vi "Temperature Limit.vi"(3 "High Limit":dbl=80.0 format="%.2f", 4 "delta t (ms)":u32=400 min=50 max=2000 step=50, 5 "Points to Acquire":i32=75 min=20 max=500) -> ()   [LabVIEW 2010]
doc: "This VI simulates the acquisition of temperature, graphs the temperature, and notifies the user if the temperature is over the limit."
panel:
  out "Over Limit":bool
  in  "Abort":bool
  out "Temperature":cluster{"Temperature":dbl, "High Limit":dbl}(graph)
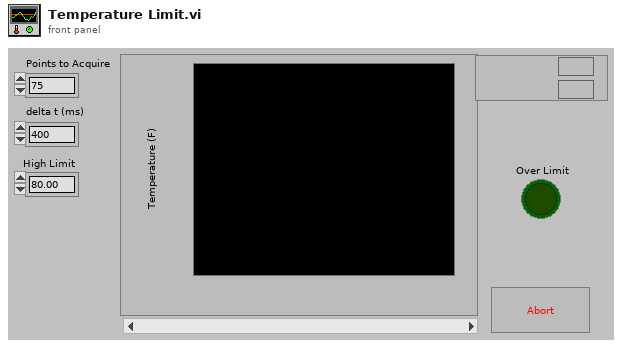
[diagram p1: front panel]
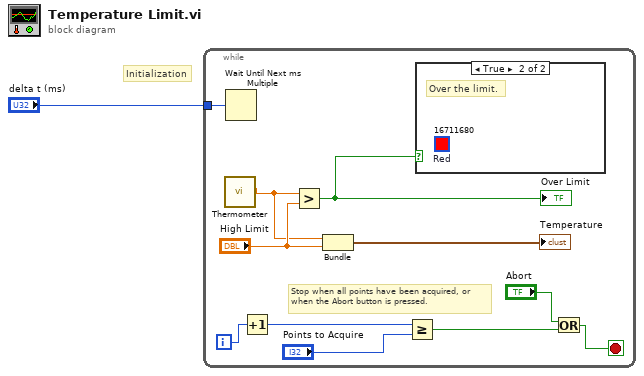
[diagram p0: block diagram]
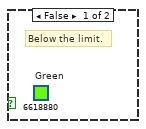
[diagram p2: hidden frame]
diagram:
  # "Initialization"
  n1 = while {
    tunnel: "delta t (ms)" -> [w4]
    i -> [w11]
    stop <- w5 stop-if-true
    # "Stop when all points have been acquired, or when the Abort button is pressed."
    n2 = call "Thermometer.vi"() -> ("Temperature"=w2:dbl)  [unwired: 10 in, 1 out]
    n3 = Wait Until Next ms Multiple(millisecond multiple=w4) -> ()  [unwired: 1 out]
    n4 = Increment(x=w11) -> (x+1=w9:i32)
    n5 = Greater?(x=w2, y="High Limit") -> (0:w3:bool)
    "Over Limit" <- w3
    n6 = Bundle("Temperature"=w2, "High Limit"="High Limit") -> (→"Temperature":cluster{"Temperature":dbl, "High Limit":dbl})  [unwired: 1 in]
    n7 = Greater Or Equal?(x=w9, y="Points to Acquire") -> (x >= y?=w7:bool)
    n8 = case shown="True" w3 {
      frame False {
        (unwired) u32 6618880  # Green
        # "Below the limit."
      }
      frame True {
        (unwired) u32 16711680  # Red
        # "Over the limit."
      }
    }
    n9 = Or(x="Abort", y=w7) -> (x .or. y?=w5:bool)
  }
